vi "Command_Goto.vi"(2 "node":string, 3 "Side":T1, 4 "Desired Position":sgl=100.0 min=0 max=100, 6 "error in":errorcluster) -> (5 "error out":errorcluster)   [LabVIEW 2012]
doc: "This will open or close the gripper to a specific position"
uses:
  <userlib>/ROSforLV/ROS/Code/SubVIs/BaxterSide.ctl
panel:
  # "Gripper position is from [0.0-100.0] [close-open]"
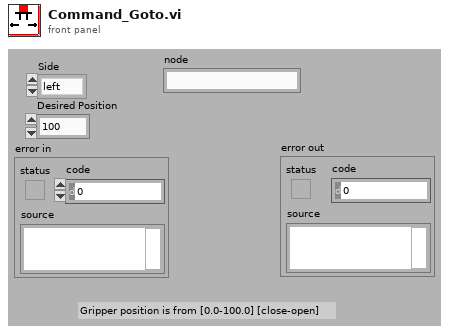
[diagram p1: front panel]
types:
  T1 = typedef "BaxterSide.ctl" = enum16{"left", "right"}
  T2 = enum16{"no_op", "set", "configure", "reboot", "reset", "calibrate", "clear_calibration", "prepare_to_grip", "grip", "release", "go", "stop"}
  T3 = typedef "TopicDef.ctl" = cluster{"Topic":string, "Type":string, "Action":T4, "Update (ms)":u16, "write queue":u16}
  T4 = typedef "_ROSDirection.ctl" = enum16{"Node", "Publisher", "Subscriber", "Service Client"}
  T5 = typedef "_ROSControl.ctl" = cluster{"topic port":u16, "Node":string, "topic":string, "type":string, "node port":u32, "error ":errorcluster, "Direction":T4, "APIs":string[], "Update (ms)":u16, "write queue":u16}
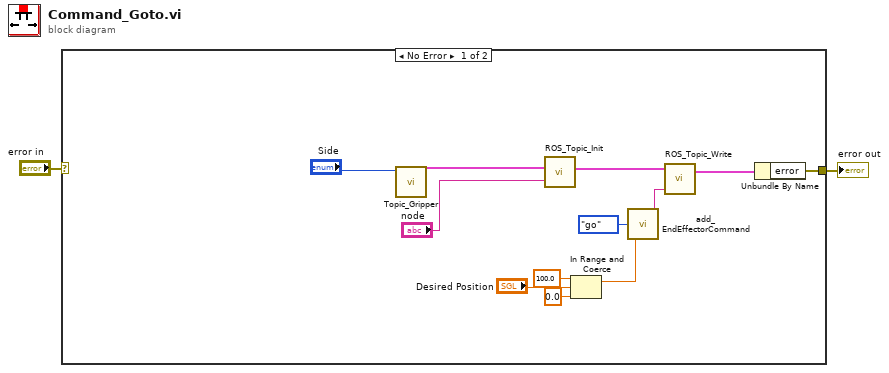
[diagram p0: block diagram]
diagram:
  n1 = case shown="No Error" "error in" {
    selector: "error in" -> [_ w15]
    tunnel: [w12 w15] -> w2
    frame No Error {
      n2 = call <userlib>:"Topic_Gripper.vi"("Side"="Side") -> ("Definitions"=w4:T3)  [unwired: 10 in]
      n3 = call <userlib>:"ROS_Topic_Init.vi"("node"="node", "Definitions"=w4) -> ("ROS out"=w14:T5)  [unwired: 1 in]
      n4 = In Range and Coerce(upper limit=sgl 100.0, x="Desired Position", lower limit=sgl 0.0) -> (coerced(x)=w6:sgl)  [unwired: 1 out]
      n5 = call <userlib>:"add_EndEffectorCommand.vi"("Position"=w6, "Commands"=T2."go") -> ("msg out"=w5:string)  [unwired: 3 in]
      n6 = call <userlib>:"ROS_Topic_Write.vi"("Msg in"=w5, "ROS in"=w14) -> ("ROS out"=w13:T5)  [unwired: 2 in]
      n7 = Unbundle By Name(w13) -> ("error"=w12:errorcluster)
    }
    frame Error {
    }
  }
  "error out" <- w2
